vi "Hysterese.vi"(8 "Abschaltung!?":sgl, 10 "soll":sgl, 11 "ist":sgl) -> (0 "Rampe":sgl, 3 "ein/aus":bool)   [LabVIEW 2020, in "Allgemein.lvlib"]
uses:
  Allgemein.lvlib
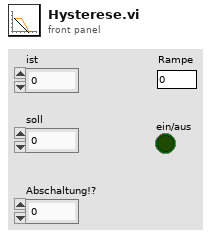
[diagram p1: front panel]
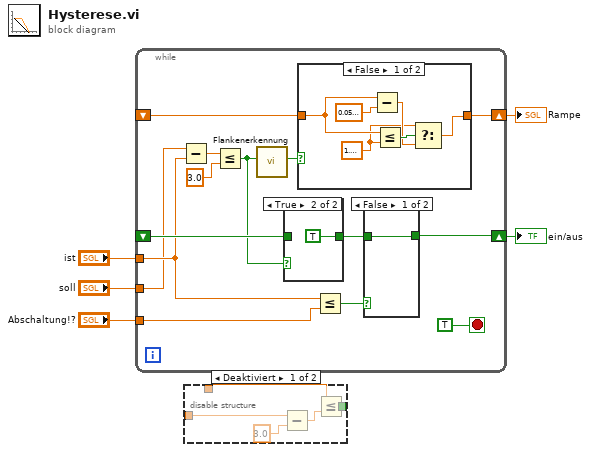
[diagram p0: block diagram]
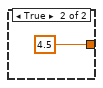
[diagram p3: hidden frame]
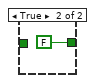
[diagram p5: hidden frame]
diagram:
  n1 = while {
    shift-right: [w17] -> w5
    shift-left: _ -> [w16]
    tunnel: "soll" -> [w7]
    tunnel: "ist" -> [w9]
    shift-right: [w13] -> w2
    shift-left: _ -> [w12]
    tunnel: "Abschaltung!?" -> [w11]
    stop <- TRUE stop-if-true
    n2 = Subtract(x=w7, y=w9) -> (x-y=w10:sgl)
    n3 = Less Or Equal?(x=w10, y=sgl 3.0 ("x")) -> (x <= y?=w6:bool)
    n4 = call "Flankenerkennung.vi"("Eingang"=w6) -> ("Steigende Flanke"=w14:bool)  [unwired: 9 in, 1 out]
    n5 = case shown="True" w6 {
      tunnel: w16 -> [w27 _]
      tunnel: [w27 TRUE ("x <= y?")] -> w15
      frame False {
      }
      frame True {
      }
    }
    n6 = case shown="False" w14 {
      tunnel: [w23 sgl 4.5] -> w13
      tunnel: w12 -> [w22 _]
      frame False {
        w21 = sgl 1.3 ("Untergrenze")
        n7 = Subtract(x=w22, y=sgl 0.05 ("Untergrenze")) -> (x-y=w24:sgl)
        n8 = Less Or Equal?(x=w22, y=w21) -> (x <= y?=w25:bool)
        n9 = Select(t=w21, s=w25, f=w24) -> (s? t:f=w23:sgl)
      }
      frame True {
      }
    }
    n10 = Less Or Equal?(x=w9, y=w11) -> (x <= y?=w18:bool)
    n11 = case shown="False" w18 {
      tunnel: [w29 FALSE ("x <= y?")] -> w17
      tunnel: w15 -> [w29 _]
      frame False {
      }
      frame True {
      }
    }
  }
  "ein/aus" <- w5
  "Rampe" <- w2
  n12 = disable-structure shown="Deaktiviert" {
    disable-tunnel: [w35 _] -> _
    disable-tunnel: _ -> [w32 _]
    disable-tunnel: _ -> [w31 _]
    frame Disabled {
      n13 = Subtract(x=w32, y=sgl 3.0) -> (x-y=w33:sgl)
      n14 = Less Or Equal?(x=w31, y=w33) -> (x <= y?=w35:bool)
    }
    frame Enabled {
    }
  }
